vi "실습 3-5 신호 Running Average.vi"() -> ()   [LabVIEW 2014]
uses:
  <vilib>/ptbypt/NI_PtbyPt.lvlib
panel:
  in  "정지":bool
  out "웨이브폼 차트":cluster{dbl, dbl, "mean":dbl}(graph)
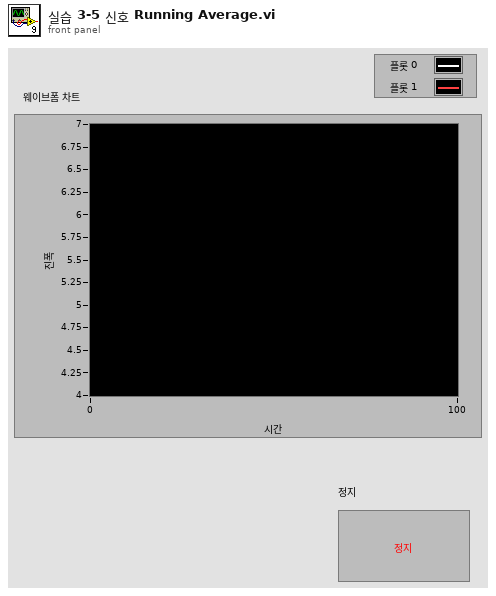
[diagram p1: front panel]
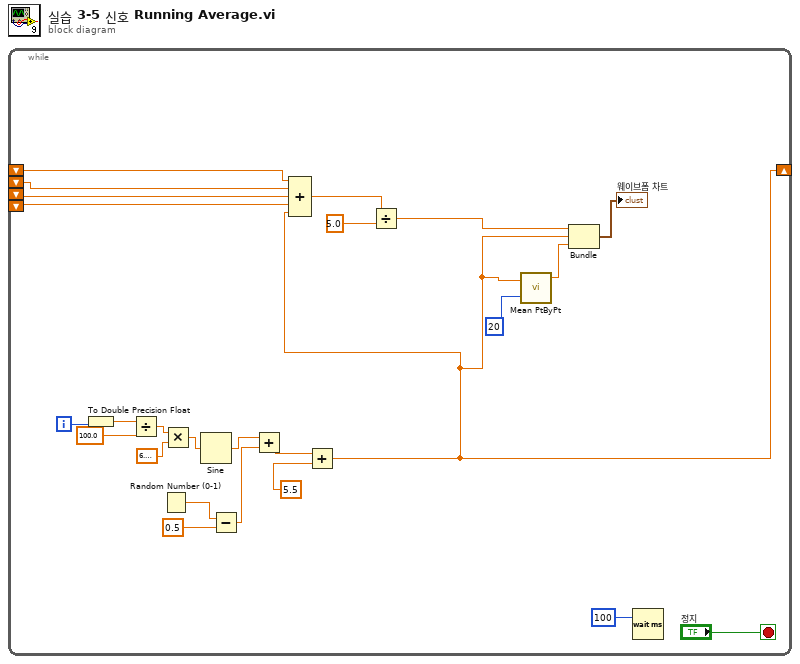
[diagram p0: block diagram]
diagram:
  n1 = while {
    shift-right: [w3] -> _
    shift-left: _ -> [w11]
    shift-left: _ -> [w8]
    shift-left: _ -> [w7]
    shift-left: _ -> [w6]
    i -> [w25]
    stop <- "정지" stop-if-true
    n2 = To Double Precision Float(number=w25) -> (double precision float=w24:dbl)
    n3 = Divide(x=w24, y=100.0) -> (x/y=w23:dbl)
    n4 = Random Number (0-1)() -> (number: 0 to 1=w14:dbl)
    n5 = Multiply(x=w23, y=6.283185307179586) -> (x*y=w22:dbl)
    n6 = Sine(x=w22) -> (sin(x)=w21:dbl)
    n7 = Subtract(x=w14, y=0.5) -> (x-y=w12:dbl)
    n8 = Add(x=w21, y=w12) -> (x+y=w20:dbl)
    n9 = Add(x=w20, y=5.5) -> (x+y=w3:dbl)
    n10 = Compound Arithmetic op=ADD(w11, w8, w7, w6, w3) -> (w10:dbl)
    n11 = Divide(x=w10, y=5.0) -> (x/y=w5:dbl)
    n12 = call <vilib>:"Mean PtByPt.vi"("x"=w3, "sample length"=20) -> ("mean"=w1:dbl)  [unwired: 2 in, 1 out]
    n13 = Bundle(w5, w3, "mean"=w1) -> (→"웨이브폼 차트":cluster{dbl, dbl, "mean":dbl})  [unwired: 1 in]
    n14 = Wait (ms)(milliseconds to wait=u32 100 ("대기 시간(ms)")) -> ()  [unwired: 1 out]
  }
